vi "basic_serial_write_and_read.vi"(0 "VISA resource name":refnum<visa-resource-name>="COM1", 1 "baud rate":u32=19200, 2 "data bits":u16=8 min=5 max=8 step=1, 3 "parity":u16(ring) items=["None", "Odd", "Even", "Mark", "Space"], 7 "flow control":u16(ring) items=["None"=0, "XON/XOFF"=1, "RTS/CTS"=2, "DTR/DSR"=4]) -> (9 "read string":string, 10 "bytes to read":u32)   [LabVIEW 2012, in "Invivo_AOTF.lvclass"]
doc: "The Basic Serial Read and Write example performs a Serial Port Read, a Serial Port Write, or a combination of these actions. The user selects the actions (read or write) on the front panel. If both are selected, the VI will write the data first, read data, and then close the VISA session that is opened to the port. This VI will wait until the specified number of bytes is received at the port. Only the number of bytes specified will be read.\n\nINSTRUCTIONS:\n1) Select the serial resource and configuration parameters (baud rate, data bits, parity, stop bits, flow control).\n2) Select the operations to be performed. \n3) Connect the serial port to your device. If no device is available, perform a loopback test by doing one of the following. Short pins 2 and 3 on a RS-232 cable or short pin 4 to pin 8 and pin 5 to pin 9 on a RS-485/422 cable. \n4) Run the VI to see the data read. (The \"read string\" will match the \"string to write\" if a loopback test was performed.)\n\nNote: The parameters set for the serial port must match the parameters of the connected instrument or device. In this example, the bytes to read parameter specifies the number of bytes that the serial port reads. If there were more bytes at the port than the number specified in bytes to read, those bytes would not be read. Also, if you specify to read more bytes than the number of bytes actually read, you might receive a timeout error message.\n\nOn the block diagram, the Configure Serial Port VI sets the configuration parameters. The front panel displays the controls used to configure the basic parameters, such as baud rate, data bits, and parity. Constants configure the other parameters the user probably does not need set. After the VISA Configure Serial Port VI opens the VISA session and configures the port, the VI passes the VISA resource name to other VIs that perform operations on that VISA resource. The VISA Write function sends a command to the serial device and the VISA Read function returns data based on the command. The VISA Close function then closes the reference to the serial device. It is important to close the reference; otherwise communication through with that port through protocols other than VISA might not be possible."
uses:
  Invivo_AOTF.lvclass
  <vilib>/Instr/_visa.llb/VISA Configure Serial Port (Instr).vi
panel:
  in  "Internal mode":bool
  in  "Line Status":bool
  in  "VISA resource name out":refnum<visa-resource-name>="COM4"
  in  "Boolean":bool=TRUE
  in  "error in (no error)":errorcluster
  in  "stop":bool
  in  "stop bits":u16(ring)=10 items=["1.0"=10, "1.5"=15, "2.0"=20]
  out "return count":u32=17
  in  "power":string="0\n0"
  in  "frequency":string="112.01"
  in  "line number":string="1"
  in  "milliseconds to wait":u32=200
  out "error out":errorcluster
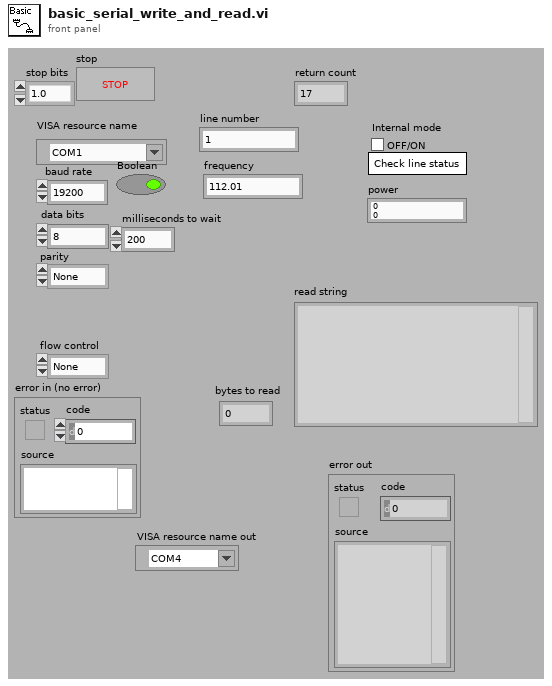
[diagram p1: front panel]
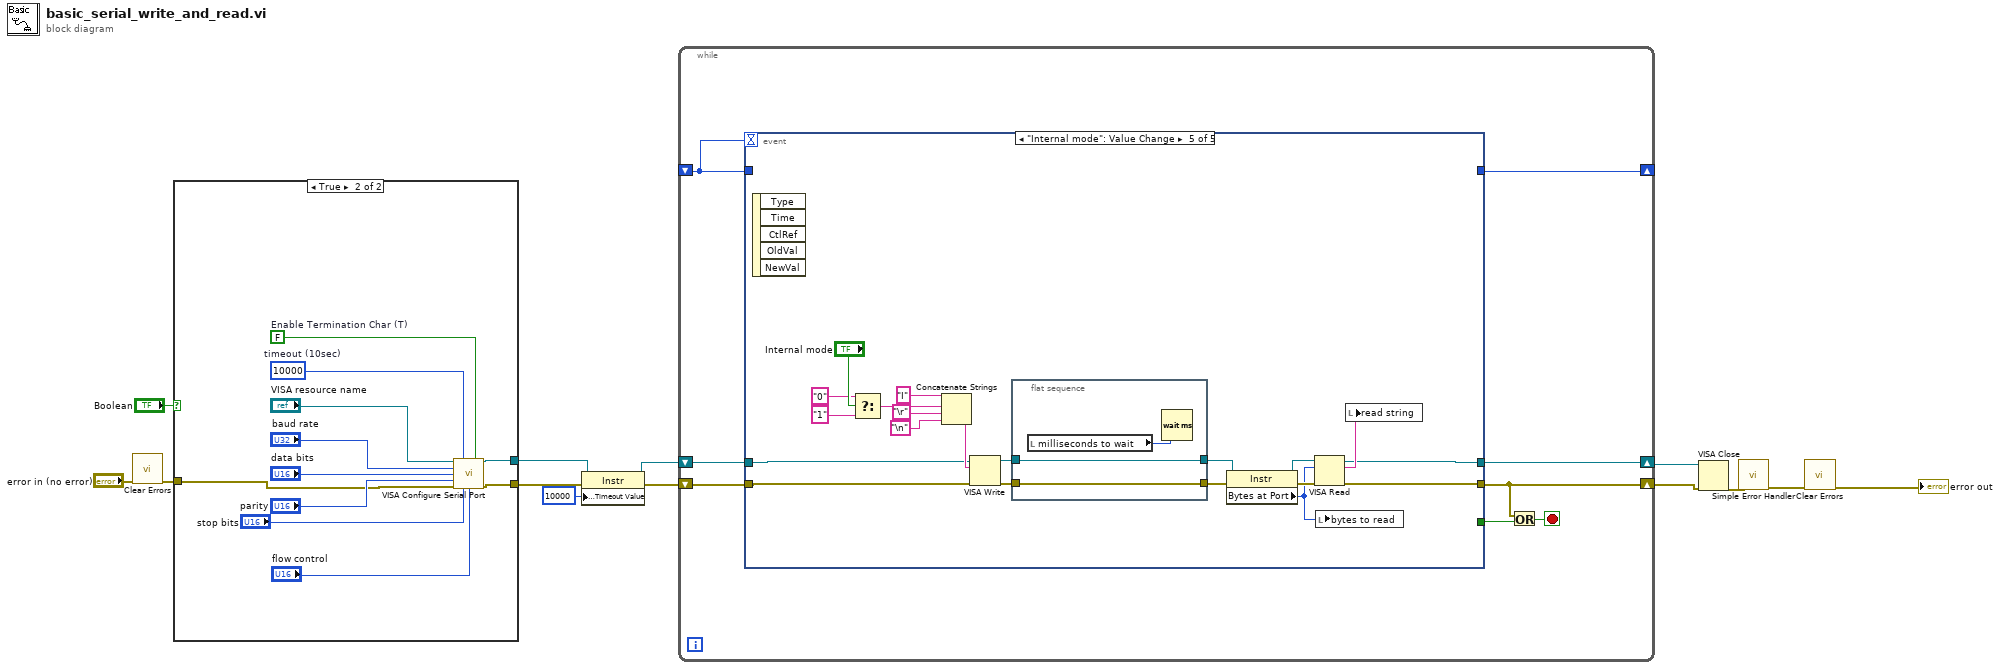
[diagram p0: block diagram]
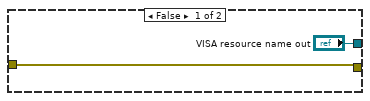
[diagram p2: hidden frame]
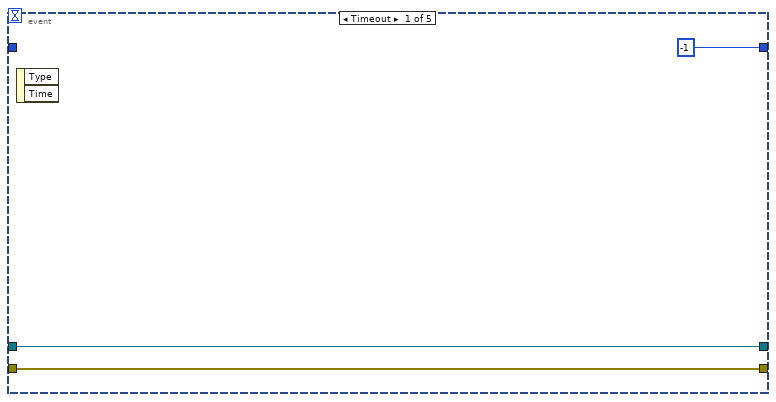
[diagram p3: hidden frame]
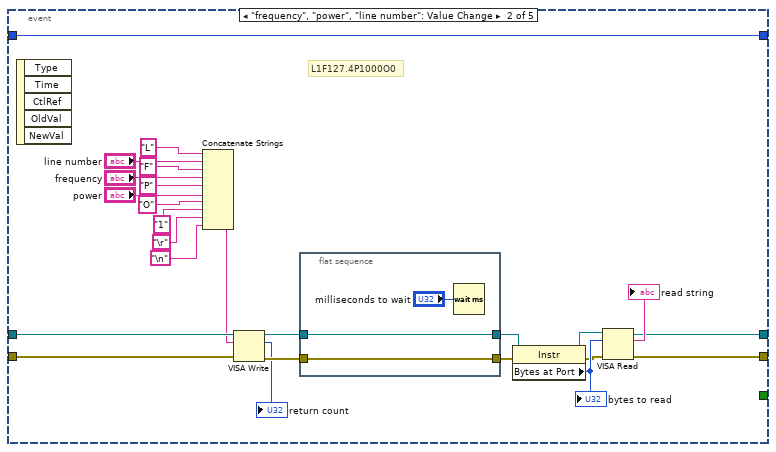
[diagram p4: hidden frame]
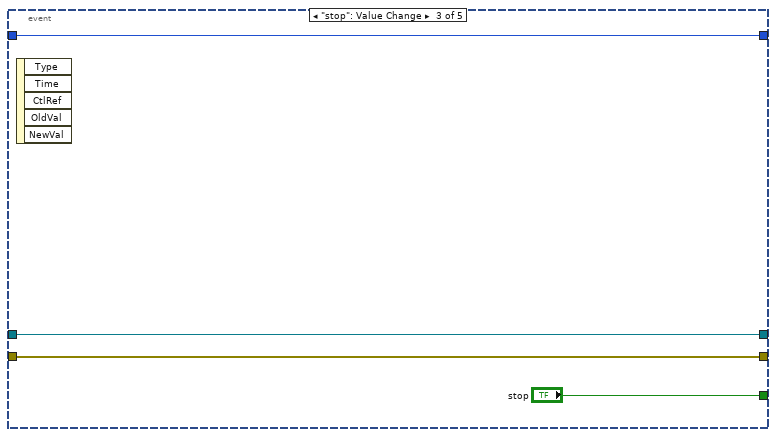
[diagram p5: hidden frame]
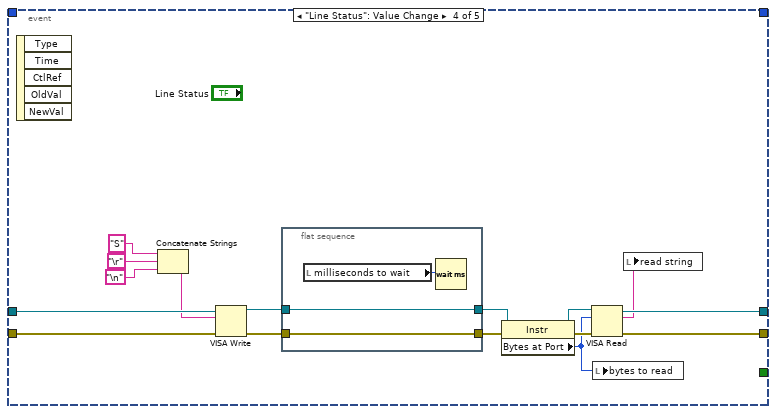
[diagram p6: hidden frame]
diagram:
  n1 = call <vilib>:"Clear Errors.vi"("error in (no error)"="error in (no error)") -> ("error out"=w10:errorcluster)  [unwired: 6 in]
  n2 = case shown="True" "Boolean" {
    tunnel: ["VISA resource name out" w18] -> w3
    tunnel: [w15 w17] -> w4
    tunnel: w10 -> [w15 w16]
    frame False {
    }
    frame True {
      w22 = FALSE  # Enable Termination Char (T)
      w23 = u32 10000  # timeout (10sec)
      n3 = call-poly "VISA Configure Serial Port"("VISA resource name"="VISA resource name", "timeout (10sec)"=w23, "Enable Termination\nChar (T)"=w22, "baud rate (9600)"="baud rate", "data bits (8)"="data bits", "parity (0:none)"="parity", "error in (no error)"=w16, "stop bits (10: 1 bit)"="stop bits", "flow control (0:none)"="flow control") -> ("VISA resource name out"=w18:refnum<visa-resource-name>, "error out"=w17:errorcluster)  [unwired: 5 in]
    }
  }
  n4 = property class="Instr"(reference=w3, error in=w4, "General Settings:Timeout Value"=u32 10000) -> (reference out=w1:refnum<visa-resource-name>, error out=w2:errorcluster)
  n5 = while {
    shift-right: [w34] -> w12
    shift-left: w1 -> [w32]
    shift-right: [w29] -> w13
    shift-left: w2 -> [w33]
    shift-right: [w28] -> _
    shift-left: _ -> [w27]
    stop <- w31 stop-if-true
    n6 = event shown="[4] \"Internal mode\": Value Change" {
      selector: _ -> [_ _ _ _ _]
      dyn-events: _ -> [_ _ _ _ _]
      timeout: w27 -> [_ _ _ _ _]
      tunnel: [w36 w44 w67 w73 w95] -> w34
      tunnel: [w35 w43 w68 w72 w94] -> w29
      tunnel: w33 -> [w35 w45 w68 w85 w96]
      tunnel: w32 -> [w36 w46 w67 w84 w97]
      tunnel: [_ _ "stop" _ _] -> w30
      tunnel: [-1 w38 w66 _ _] -> w28
      tunnel: w27 -> [_ w38 w66 _ _]
      event Timeout {
        n7 = event-data() -> ()  [unwired: 1 in, 2 out]
      }
      event "frequency", "power", "line number": Value Change {
        # "L1F127.4P1000O0"
        n8 = event-data() -> ()  [unwired: 1 in, 5 out]
        n9 = Concatenate Strings("L", "line number", "F" ("string"), "frequency", "P" ("string"), "power", "O" ("string"), "1" ("On/Off"), "\r", "\n") -> (w40:string)
        n10 = VISA Write(VISA resource name=w46, write buffer=w40, error in (no error)=w45) -> (VISA resource name out=w60:refnum<visa-resource-name>, return count=→"return count":u32, error out=w62:errorcluster)
        n11 = flat-sequence {
          tunnel: [w65] -> w61
          tunnel: w62 -> [w65]
          tunnel: [w64] -> w59
          tunnel: w60 -> [w64]
          frame #0 {
            n12 = Wait (ms)(milliseconds to wait="milliseconds to wait") -> ()  [unwired: 1 out]
          }
        }
        n13 = property class="Instr"(reference=w59, error in=w61) -> (reference out=w39:refnum<visa-resource-name>, error out=w56:errorcluster, "Bytes at Port"=w57:u32)
        "bytes to read" <- w57
        n14 = VISA Read(VISA resource name=w39, byte count=w57, error in (no error)=w56) -> (VISA resource name out=w44:refnum<visa-resource-name>, read buffer=→"read string":string, error out=w43:errorcluster)  [unwired: 1 out]
      }
      event "stop": Value Change {
        n15 = event-data() -> ()  [unwired: 1 in, 5 out]
      }
      event "Line Status": Value Change {
        n16 = event-data() -> ()  [unwired: 1 in, 5 out]
        n17 = Concatenate Strings("S" ("On/Off"), "\r", "\n") -> (w80:string)
        n18 = VISA Write(VISA resource name=w84, write buffer=w80, error in (no error)=w85) -> (VISA resource name out=w78:refnum<visa-resource-name>, error out=w79:errorcluster)  [unwired: 1 out]
        n19 = flat-sequence {
          tunnel: [w88] -> w74
          tunnel: w79 -> [w88]
          tunnel: [w87] -> w75
          tunnel: w78 -> [w87]
          frame #0 {
            n20 = local read "milliseconds to wait"() -> (w86:u32)
            n21 = Wait (ms)(milliseconds to wait=w86) -> ()  [unwired: 1 out]
          }
        }
        n22 = property class="Instr"(reference=w75, error in=w74) -> (reference out=w77:refnum<visa-resource-name>, error out=w76:errorcluster, "Bytes at Port"=w70:u32)
        n23 = VISA Read(VISA resource name=w77, byte count=w70, error in (no error)=w76) -> (VISA resource name out=w73:refnum<visa-resource-name>, read buffer=w71:string, error out=w72:errorcluster)  [unwired: 1 out]
        n24 = local write "bytes to read"(w70) -> ()
        n25 = local write "read string"(w71) -> ()
      }
      event "Internal mode": Value Change {
        n26 = event-data() -> ()  [unwired: 1 in, 5 out]
        n27 = Select(t="0" ("On/Off"), s="Internal mode", f="1" ("On/Off")) -> (s? t:f=w89:string)
        n28 = Concatenate Strings("I" ("On/Off"), w89, "\r", "\n") -> (w106:string)
        n29 = VISA Write(VISA resource name=w97, write buffer=w106, error in (no error)=w96) -> (VISA resource name out=w104:refnum<visa-resource-name>, error out=w105:errorcluster)  [unwired: 1 out]
        n30 = flat-sequence {
          tunnel: [w111] -> w100
          tunnel: w105 -> [w111]
          tunnel: [w110] -> w101
          tunnel: w104 -> [w110]
          frame #0 {
            n31 = local read "milliseconds to wait"() -> (w109:u32)
            n32 = Wait (ms)(milliseconds to wait=w109) -> ()  [unwired: 1 out]
          }
        }
        n33 = property class="Instr"(reference=w101, error in=w100) -> (reference out=w103:refnum<visa-resource-name>, error out=w102:errorcluster, "Bytes at Port"=w98:u32)
        n34 = VISA Read(VISA resource name=w103, byte count=w98, error in (no error)=w102) -> (VISA resource name out=w95:refnum<visa-resource-name>, read buffer=w99:string, error out=w94:errorcluster)  [unwired: 1 out]
        n35 = local write "bytes to read"(w98) -> ()
        n36 = local write "read string"(w99) -> ()
      }
    }
    n37 = Or(x=w29, y=w30) -> (x .or. y?=w31:bool)
  }
  n38 = VISA Close(VISA resource name=w12, error in (no error)=w13) -> (error out=w11:errorcluster)
  n39 = call <vilib>:"Simple Error Handler.vi"("error in (no error)"=w11) -> ("error out"=w8:errorcluster)  [unwired: 4 in, 4 out]
  n40 = call <vilib>:"Clear Errors.vi"("error in (no error)"=w8) -> ("error out"=→"error out":errorcluster)  [unwired: 6 in]
